vi "TabVisibilityControl.vi"(8 "error in (no error)":errorcluster, 10 "Tab Control 2":refnum<vi>, 11 "Tab control":cluster{"visible":bool, "Tab name":string}[](array[cluster])=[{"visible"=FALSE, "Tab name"="Experiment Controller"}, {"visible"=FALSE, "Tab name"="Pulse Programming"}, {"visible"=FALSE, "Tab name"="Pulse Sequence"}, {"visible"=FALSE, "Tab name"="DDS Boards"}, {"visible"=FALSE, "Tab name"="Calypso"}, {"visible"=FALSE, "Tab name"="Digital/Analog"}, {"visible"=FALSE, "Tab name"="Cryo DC"}]) -> (0 "error out":errorcluster, 3 "Running VIs ref":refnum<vi>[](array[refnum]))   [LabVIEW 2019]
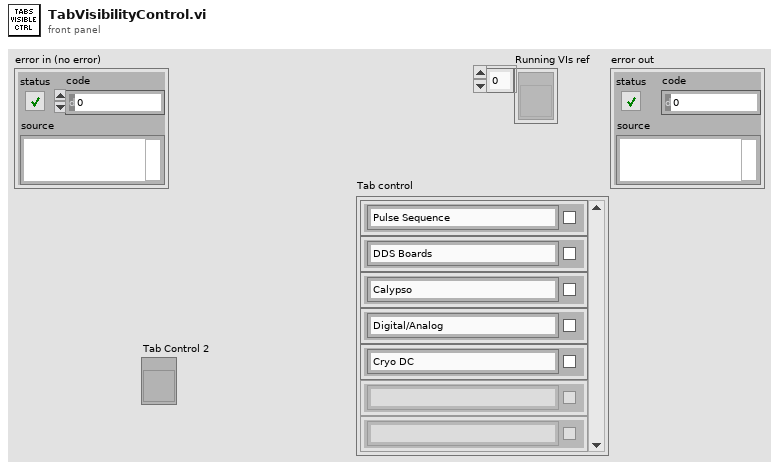
[diagram p1: front panel]
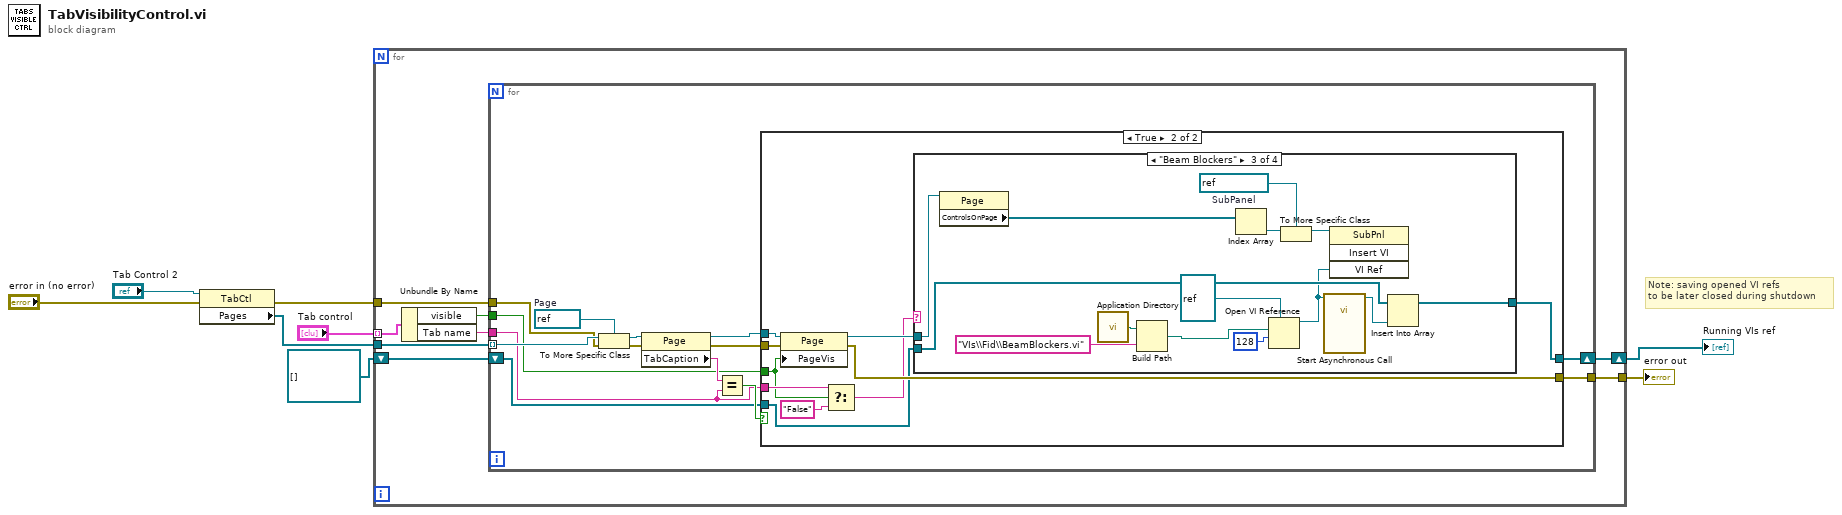
[diagram p0: block diagram]
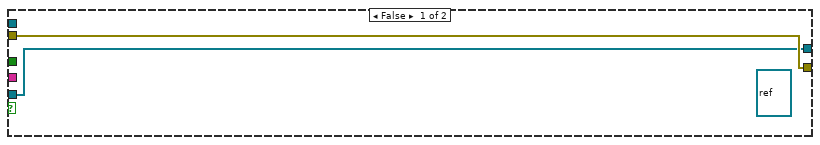
[diagram p2: hidden frame]
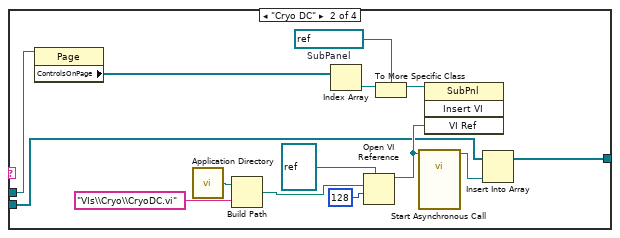
[diagram p4: hidden frame]
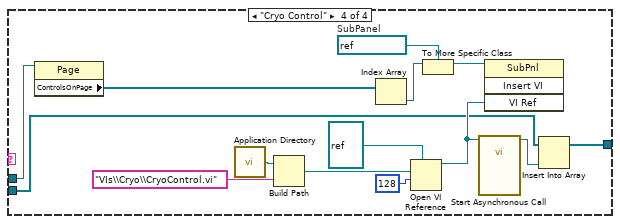
[diagram p5: hidden frame]
diagram:
  # "Note: saving opened VI refs\nto be later closed during shutdown"
  n1 = property class="TabCtl"(reference="Tab Control 2", error in="error in (no error)") -> (error out=w5:errorcluster, "Pages"=w6:refnum<vi>[])  [unwired: 1 out]
  n2 = for {
    tunnel: "Tab control" -> [w15] mode=indexing
    tunnel: w6 -> [w16]
    tunnel: w5 -> [w12]
    tunnel: [w11] -> w4
    shift-right: [w9] -> w1
    shift-left: refnum<vi>[] [] -> [w10]
    n3 = Unbundle By Name(w15) -> ("visible"=w13:bool, "Tab name"=w14:string)
    n4 = for {
      tunnel: w16 -> [w30] mode=indexing
      tunnel: w14 -> [w19]
      tunnel: w13 -> [w24]
      tunnel: w12 -> [w23]
      tunnel: [w20] -> w11
      shift-right: [w17] -> w9
      shift-left: w10 -> [w18]
      w28 = refnum<vi> refnum  # Page
      n5 = To More Specific Class(target class=w28, reference=w30, error in=w23) -> (specific class reference=w29:refnum<vi>, error out=w22:errorcluster)
      n6 = property class="Page"(reference=w29, error in=w22) -> (reference out=w25:refnum<vi>, error out=w21:errorcluster, "TabCaption"=w27:string)
      n7 = Equal?(x=w27, y=w19) -> (x = y?=w26:bool)
      n8 = case shown="True" w26 {
        tunnel: w25 -> [_ w42]
        tunnel: w24 -> [_ w37]
        tunnel: w21 -> [w32 w41]
        tunnel: [w32 w40] -> w20
        tunnel: w19 -> [_ w38]
        tunnel: w18 -> [w31 w34]
        tunnel: [w31 w33] -> w17
        frame False {
          (unwired) refnum<vi> refnum ("type specifier VI Refnum (for type only)")
        }
        frame True {
          n9 = property class="Page"(reference=w42, error in=w41, "PageVis"=w37) -> (reference out=w39:refnum<vi>, error out=w40:errorcluster)
          n10 = Select(t=w38, s=w37, f="False") -> (s? t:f=w35:string)
          n11 = case shown="\"Beam Blockers\"" w35 {
            tunnel: w39 -> [_ w51 w71 w77]
            tunnel: w34 -> [w43 w46 w70 w73]
            tunnel: [w43 w44 w69 w72] -> w33
            frame "False", Default {
            }
            frame "Cryo DC" {
              w48 = refnum<vi> refnum  # SubPanel
              n12 = property class="Page"(reference=w51) -> ("ControlsOnPage"=w50:refnum<vi>[])  [unwired: 1 in, 2 out]
              n13 = call <vilib>:"Application Directory.vi"() -> ("Application Directory"=w57:path)
              n14 = Build Path(base path=w57, name or relative path="VIs\\Cryo\\CryoDC.vi") -> (appended path=w55:path)
              n15 = Index Array(array=w50) -> (element=w49:refnum<vi>)  [unwired: 1 in]
              n16 = Open VI Reference(type specifier VI Refnum (for type only)=refnum<vi> refnum, vi path=w55, options=128) -> (vi reference=w52:refnum<vi>)  [unwired: 3 in, 1 out]
              n17 = To More Specific Class(target class=w48, reference=w49) -> (specific class reference=w47:refnum<vi>)  [unwired: 1 in, 1 out]
              n18 = call-by-ref "Start Asynchronous Call"(reference=w52) -> (reference out=w45:refnum<vi>)  [unwired: 2 in, 1 out]
              n19 = invoke on="Invoke Node" class="SubPnl" method="Insert VI"(reference=w47, "VI Ref"=w52) -> ()  [unwired: 2 in, 4 out]
              n20 = Insert Into Array(array=w46, new element=w45) -> (w44:refnum<vi>[])  [unwired: 1 in]
            }
            frame "Beam Blockers" {
              w61 = refnum<vi> refnum  # SubPanel
              n21 = property class="Page"(reference=w71) -> ("ControlsOnPage"=w63:refnum<vi>[])  [unwired: 1 in, 2 out]
              n22 = call <vilib>:"Application Directory.vi"() -> ("Application Directory"=w68:path)
              n23 = Build Path(base path=w68, name or relative path="VIs\\Fid\\BeamBlockers.vi") -> (appended path=w66:path)
              n24 = Index Array(array=w63) -> (element=w62:refnum<vi>)  [unwired: 1 in]
              n25 = Open VI Reference(type specifier VI Refnum (for type only)=refnum<vi> refnum, vi path=w66, options=128) -> (vi reference=w64:refnum<vi>)  [unwired: 3 in, 1 out]
              n26 = To More Specific Class(target class=w61, reference=w62) -> (specific class reference=w60:refnum<vi>)  [unwired: 1 in, 1 out]
              n27 = call-by-ref "Start Asynchronous Call"(reference=w64) -> (reference out=w59:refnum<vi>)  [unwired: 13 in, 1 out]
              n28 = invoke on="Invoke Node" class="SubPnl" method="Insert VI"(reference=w60, "VI Ref"=w64) -> ()  [unwired: 2 in, 4 out]
              n29 = Insert Into Array(array=w70, new element=w59) -> (w69:refnum<vi>[])  [unwired: 1 in]
            }
            frame "Cryo Control" {
              w78 = refnum<vi> refnum  # SubPanel
              n30 = property class="Page"(reference=w77) -> ("ControlsOnPage"=w80:refnum<vi>[])  [unwired: 1 in, 2 out]
              n31 = call <vilib>:"Application Directory.vi"() -> ("Application Directory"=w85:path)
              n32 = Build Path(base path=w85, name or relative path="VIs\\Cryo\\CryoControl.vi") -> (appended path=w83:path)
              n33 = Index Array(array=w80) -> (element=w79:refnum<vi>)  [unwired: 1 in]
              n34 = Open VI Reference(type specifier VI Refnum (for type only)=refnum<vi> refnum, vi path=w83, options=128) -> (vi reference=w76:refnum<vi>)  [unwired: 3 in, 1 out]
              n35 = To More Specific Class(target class=w78, reference=w79) -> (specific class reference=w75:refnum<vi>)  [unwired: 1 in, 1 out]
              n36 = call-by-ref "Start Asynchronous Call"(reference=w76) -> (reference out=w74:refnum<vi>)  [unwired: 13 in, 1 out]
              n37 = invoke on="Invoke Node" class="SubPnl" method="Insert VI"(reference=w75, "VI Ref"=w76) -> ()  [unwired: 2 in, 4 out]
              n38 = Insert Into Array(array=w73, new element=w74) -> (w72:refnum<vi>[])  [unwired: 1 in]
            }
          }
        }
      }
    }
  }
  "error out" <- w4
  "Running VIs ref" <- w1
